vi "sample_calibration_process_centroids.vi"(8 "Error In":errorcluster, 10 "Right Centroids":dbl[][](array[numeric]), 11 "Left Centroids":dbl[][](array[numeric])) -> (0 "Error Out":errorcluster, 3 "Results":T1)   [LabVIEW 2019]
uses:
  centroid_difference_cluster_typedef.ctl
  <vilib>/Analysis/baseanly.llb/Mean (DBL).vi
  <vilib>/Analysis/NI_AALBase.lvlib
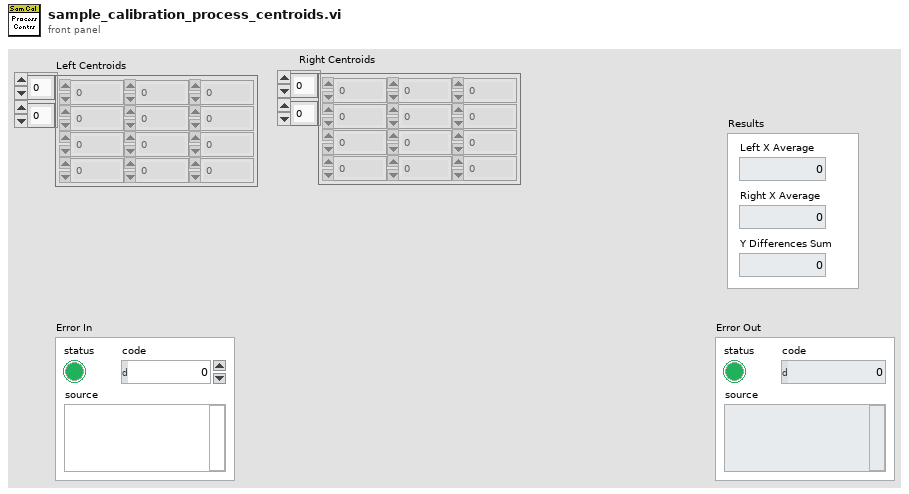
[diagram p1: front panel]
types:
  T1 = typedef "centroid_difference_cluster_typedef.ctl" = cluster{"Left X Average":dbl, "Right X Average":dbl, "Y Differences Sum":dbl}
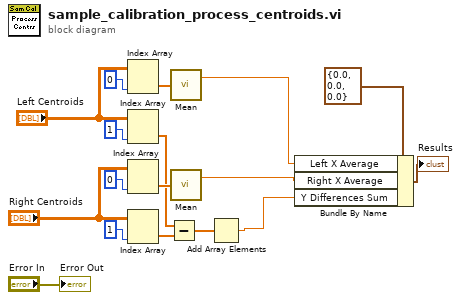
[diagram p0: block diagram]
diagram:
  n1 = Index Array(array="Left Centroids", index (col)=0 ("disabled index (col)")) -> (element=w16:dbl[])  [unwired: 1 in]
  n2 = Index Array(array="Left Centroids", index (col)=1 ("disabled index (col)")) -> (element=w9:dbl[])  [unwired: 1 in]
  n3 = Index Array(array="Right Centroids", index (col)=0 ("disabled index (col)")) -> (element=w15:dbl[])  [unwired: 1 in]
  n4 = Index Array(array="Right Centroids", index (col)=1 ("disabled index (col)")) -> (element=w8:dbl[])  [unwired: 1 in]
  n5 = Subtract(x=w9, y=w8) -> (x-y=w7:dbl[])
  n6 = call-poly <vilib>:"Mean.vi"("X"=w16) -> ("mean"=w1:dbl)  [unwired: 1 out]
  n7 = call-poly <vilib>:"Mean.vi"("X"=w15) -> ("mean"=w2:dbl)  [unwired: 1 out]
  n8 = Add Array Elements(numeric array=w7) -> (sum=w3:dbl)
  n9 = Bundle By Name(cluster=T1 {"Left X Average"=0.0, "Right X Average"=0.0, "Y Differences Sum"=0.0} ("Results"), "Left X Average"=w1, "Right X Average"=w2, "Y Differences Sum"=w3) -> (→"Results":T1)
  "Error Out" <- "Error In"
